vi "EncAlg.vi"(10 "EnValIn":dbl[](array[numeric]), 11 "element":T1) -> (0 "VelValOut":dbl[](array[numeric]), 1 "0, 1":i16, 2 "logical AND":bool)   [LabVIEW 2019]
panel:
  out "x":dbl
  out "y":dbl
  out "o":dbl
  out "Sense":dbl
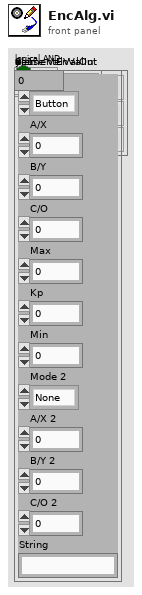
[diagram p1: front panel]
types:
  T1 = cluster{"Mode":enum16{"Button", "Encoder", "Delay", "IR Stop", "Line Stop"}, "A/X":dbl, "B/Y":dbl, "C/O":dbl, "Max":dbl, "Kp":dbl, "Min":dbl, "Mode 2":enum16{"None", "IR Stabilize", "Line Stabilize", "Encoder", "IR Stop", "Servo"}, "A/X 2":dbl, "B/Y 2":dbl, "C/O 2":dbl, "String":string}
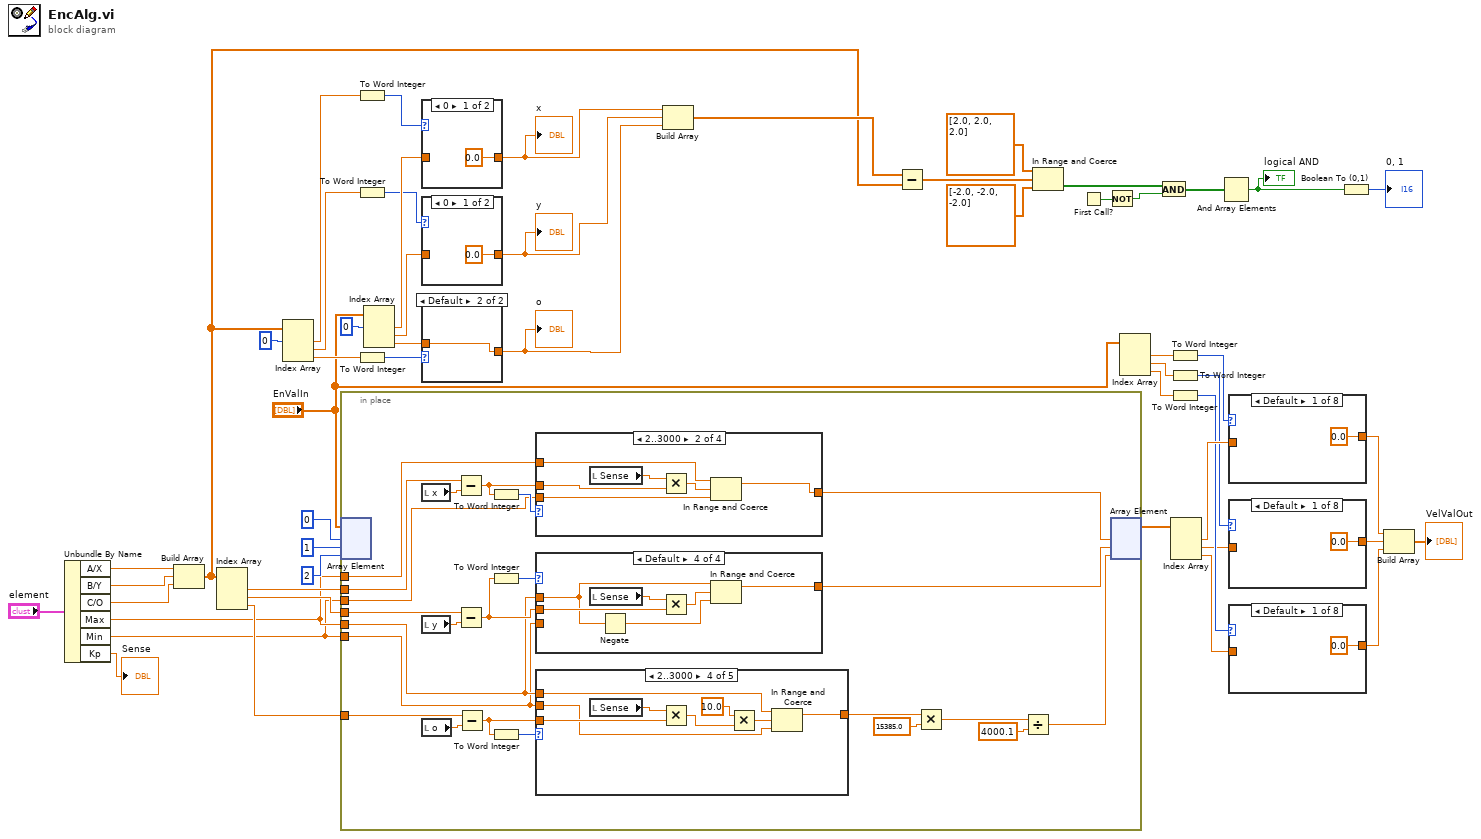
[diagram p0: block diagram]
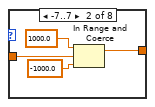
[diagram p2: hidden frame]
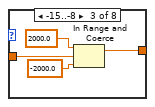
[diagram p3: hidden frame]
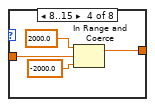
[diagram p4: hidden frame]
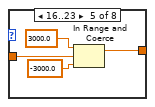
[diagram p5: hidden frame]
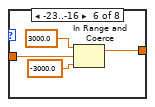
[diagram p6: hidden frame]
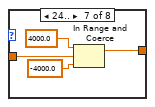
[diagram p7: hidden frame]
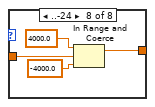
[diagram p8: hidden frame]
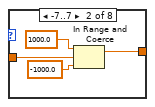
[diagram p9: hidden frame]
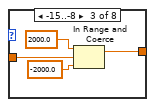
[diagram p10: hidden frame]
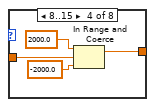
[diagram p11: hidden frame]
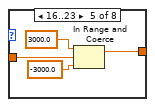
[diagram p12: hidden frame]
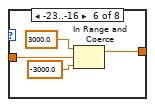
[diagram p13: hidden frame]
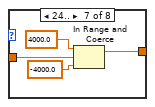
[diagram p14: hidden frame]
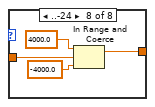
[diagram p15: hidden frame]
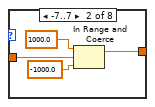
[diagram p16: hidden frame]
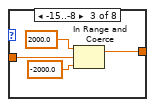
[diagram p17: hidden frame]
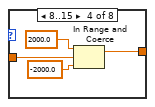
[diagram p18: hidden frame]
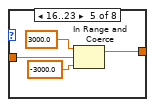
[diagram p19: hidden frame]
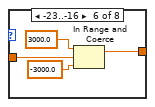
[diagram p20: hidden frame]
diagram:
  n1 = Unbundle By Name("element") -> ("A/X"=w47:dbl, "B/Y"=w46:dbl, "C/O"=w45:dbl, "Max"=w44:dbl, "Min"=w43:dbl, "Kp"=→"Sense":dbl)
  n2 = Build Array(w47, w46, w45) -> (w1:dbl[])
  n3 = Index Array(array=w1) -> (element #1=w49:dbl, element #2=w53:dbl, element #3=w48:dbl)  [unwired: 3 in]
  n4 = Index Array(array=w1, index #1=0 ("index")) -> (element #1=w39:dbl, element #2=w38:dbl, element #3=w37:dbl)  [unwired: 2 in]
  n5 = in-place {
    in-place-border: w53 -> [w76]
    in-place-border: w49 -> [w75]
    in-place-border: w48 -> [w74]
    in-place-border: w44 -> [w68]
    in-place-border: w43 -> [w67]
    in-place-border: w44 -> [w64]
    in-place-border: w43 -> [w63]
    n6 = in-place-array #1("EnValIn", 0, 1, 2) -> ()  [unwired: 3 out]
    n7 = local read "x"() -> (w54:dbl)
    n8 = local read "y"() -> (w55:dbl)
    n9 = local read "o"() -> (w56:dbl)
    n10 = Subtract(x=w75, y=w54) -> (x-y=w66:dbl)
    n11 = Subtract(x=w76, y=w55) -> (x-y=w65:dbl)
    n12 = Subtract(x=w74, y=w56) -> (x-y=w62:dbl)
    n13 = To Word Integer(number=w66) -> (16bit integer=w69:i16)
    n14 = To Word Integer(number=w65) -> (16bit integer=w70:i16)
    n15 = To Word Integer(number=w62) -> (16bit integer=w71:i16)
    n16 = case shown="2..3000" w69 {
      tunnel: w66 -> [_ w138 w146 w152]
      tunnel: [0.0 ("x") w139 w147 w153] -> w73
      tunnel: w68 -> [_ w137 w145 w151]
      tunnel: w67 -> [_ w136 w143 _]
      frame -1..1 {
      }
      frame 2..3000 {
        n17 = local read "Sense"() -> (w135:dbl)
        n18 = Multiply(x=w135, y=w138) -> (x*y=w140:dbl)
        n19 = In Range and Coerce(upper limit=w137, x=w140, lower limit=w136) -> (coerced(x)=w139:dbl)  [unwired: 1 out]
      }
      frame -3000..-2 {
        n20 = local read "Sense"() -> (w141:dbl)
        n21 = Negate(x=w143) -> (-x=w144:dbl)
        n22 = Negate(x=w145) -> (-x=w142:dbl)
        n23 = Multiply(x=w141, y=w146) -> (x*y=w148:dbl)
        n24 = In Range and Coerce(upper limit=w142, x=w148, lower limit=w144) -> (coerced(x)=w147:dbl)  [unwired: 1 out]
      }
      frame Default {
        n25 = local read "Sense"() -> (w149:dbl)
        n26 = Negate(x=w151) -> (-x=w150:dbl)
        n27 = Multiply(x=w149, y=w152) -> (x*y=w154:dbl)
        n28 = In Range and Coerce(upper limit=w151, x=w154, lower limit=w150) -> (coerced(x)=w153:dbl)  [unwired: 1 out]
      }
    }
    n29 = case shown="Default" w70 {
      tunnel: w65 -> [_ w117 w125 w131]
      tunnel: [0.0 ("x") w118 w126 w132] -> w72
      tunnel: w64 -> [_ w116 w121 w129]
      tunnel: w63 -> [_ w115 w122 _]
      frame -1..1 {
      }
      frame 2..3000 {
        n30 = local read "Sense"() -> (w114:dbl)
        n31 = Multiply(x=w114, y=w117) -> (x*y=w119:dbl)
        n32 = In Range and Coerce(upper limit=w116, x=w119, lower limit=w115) -> (coerced(x)=w118:dbl)  [unwired: 1 out]
      }
      frame -3000..-2 {
        n33 = local read "Sense"() -> (w120:dbl)
        n34 = Negate(x=w122) -> (-x=w123:dbl)
        n35 = Negate(x=w121) -> (-x=w124:dbl)
        n36 = Multiply(x=w120, y=w125) -> (x*y=w127:dbl)
        n37 = In Range and Coerce(upper limit=w124, x=w127, lower limit=w123) -> (coerced(x)=w126:dbl)  [unwired: 1 out]
      }
      frame Default {
        n38 = local read "Sense"() -> (w128:dbl)
        n39 = Negate(x=w129) -> (-x=w130:dbl)
        n40 = Multiply(x=w128, y=w131) -> (x*y=w133:dbl)
        n41 = In Range and Coerce(upper limit=w129, x=w133, lower limit=w130) -> (coerced(x)=w132:dbl)  [unwired: 1 out]
      }
    }
    n42 = case shown="2..3000" w71 {
      tunnel: w62 -> [w81 w90 _ w100 w110]
      tunnel: [w82 w91 0.0 ("x") w101 w111] -> w58
      tunnel: w64 -> [w78 w86 _ w98 w108]
      tunnel: w63 -> [_ w87 _ w97 w107]
      frame -1, 1 {
        n43 = local read "Sense"() -> (w79:dbl)
        n44 = Negate(x=w78) -> (-x=w77:dbl)
        n45 = Multiply(x=w81, y=w79) -> (x*y=w80:dbl)
        n46 = Multiply(x=10.0, y=w80) -> (x*y=w84:dbl)
        n47 = In Range and Coerce(upper limit=w78, x=w84, lower limit=w77) -> (coerced(x)=w82:dbl)  [unwired: 1 out]
      }
      frame Default {
        n48 = local read "Sense"() -> (w88:dbl)
        n49 = Negate(x=w86) -> (-x=w85:dbl)
        n50 = Multiply(x=w90, y=w88) -> (x*y=w89:dbl)
        n51 = Multiply(x=10.0, y=w89) -> (x*y=w93:dbl)
        n52 = In Range and Coerce(upper limit=w87, x=w93, lower limit=w85) -> (coerced(x)=w91:dbl)  [unwired: 1 out]
      }
      frame 0 {
      }
      frame 2..3000 {
        n53 = local read "Sense"() -> (w99:dbl)
        n54 = Multiply(x=w99, y=w100) -> (x*y=w102:dbl)
        n55 = Multiply(x=10.0, y=w102) -> (x*y=w96:dbl)
        n56 = In Range and Coerce(upper limit=w98, x=w96, lower limit=w97) -> (coerced(x)=w101:dbl)  [unwired: 1 out]
      }
      frame -3000..-2 {
        n57 = local read "Sense"() -> (w109:dbl)
        n58 = Negate(x=w107) -> (-x=w105:dbl)
        n59 = Negate(x=w108) -> (-x=w106:dbl)
        n60 = Multiply(x=w109, y=w110) -> (x*y=w112:dbl)
        n61 = Multiply(x=10.0, y=w112) -> (x*y=w104:dbl)
        n62 = In Range and Coerce(upper limit=w106, x=w104, lower limit=w105) -> (coerced(x)=w111:dbl)  [unwired: 1 out]
      }
    }
    n63 = Multiply(x=w58, y=15385.0) -> (x*y=w61:dbl)
    n64 = Divide(x=w61, y=4000.1) -> (x/y=w57:dbl)
    n65 = in-place-array #1(w73, w72, w57) -> (w33:dbl[])  [unwired: 3 out]
  }
  n66 = To Word Integer(number=w39) -> (16bit integer=w18:i16)
  n67 = To Word Integer(number=w38) -> (16bit integer=w16:i16)
  n68 = To Word Integer(number=w37) -> (16bit integer=w15:i16)
  n69 = Index Array(array="EnValIn", index #1=0 ("index")) -> (element #1=w17:dbl, element #2=w36:dbl, element #3=w35:dbl)  [unwired: 2 in]
  n70 = case shown="0" w18 {
    tunnel: [0.0 w156] -> w5
    tunnel: w17 -> [_ w156]
    frame 0 {
    }
    frame Default {
    }
  }
  "x" <- w5
  n71 = case shown="0" w16 {
    tunnel: [0.0 w158] -> w4
    tunnel: w36 -> [_ w158]
    frame 0 {
    }
    frame Default {
    }
  }
  "y" <- w4
  n72 = case shown="Default" w15 {
    tunnel: [0.0 w160] -> w3
    tunnel: w35 -> [_ w160]
    frame 0 {
    }
    frame Default {
    }
  }
  "o" <- w3
  n73 = Build Array(w5, w4, w3) -> (w2:dbl[])
  n74 = Subtract(x=w2, y=w1) -> (x-y=w14:dbl[])
  n75 = In Range and Coerce(upper limit=dbl[] [2.0, 2.0, 2.0], x=w14, lower limit=dbl[] [-2.0, -2.0, -2.0]) -> (In Range?=w11:bool[])  [unwired: 1 out]
  n76 = First Call?() -> (First Call?: T/F=w10:bool)
  n77 = Not(x=w10) -> (.not. x?=w9:bool)
  n78 = Index Array(array="EnValIn") -> (element #1=w30:dbl, element #2=w27:dbl, element #3=w26:dbl)  [unwired: 3 in]
  n79 = And(x=w11, y=w9) -> (x .and. y?=w8:bool[])
  n80 = To Word Integer(number=w30) -> (16bit integer=w29:i16)
  n81 = To Word Integer(number=w27) -> (16bit integer=w25:i16)
  n82 = To Word Integer(number=w26) -> (16bit integer=w24:i16)
  n83 = Index Array(array=w33) -> (element #1=w32:dbl, element #2=w23:dbl, element #3=w22:dbl)  [unwired: 3 in]
  n84 = And Array Elements(Boolean array=w8) -> (logical AND=w7:bool)
  "logical AND" <- w7
  n85 = case shown="Default" w29 {
    tunnel: w32 -> [_ w164 w168 w172 w176 w180 w184 w188]
    tunnel: [0.0 ("upper limit") w162 w166 w170 w174 w178 w182 w186] -> w28
    frame Default {
    }
    frame -7..7 {
      n86 = In Range and Coerce(upper limit=1000.0, x=w164, lower limit=-1000.0) -> (coerced(x)=w162:dbl)  [unwired: 1 out]
    }
    frame -15..-8 {
      n87 = In Range and Coerce(upper limit=2000.0, x=w168, lower limit=-2000.0) -> (coerced(x)=w166:dbl)  [unwired: 1 out]
    }
    frame 8..15 {
      n88 = In Range and Coerce(upper limit=2000.0, x=w172, lower limit=-2000.0) -> (coerced(x)=w170:dbl)  [unwired: 1 out]
    }
    frame 16..23 {
      n89 = In Range and Coerce(upper limit=3000.0, x=w176, lower limit=-3000.0) -> (coerced(x)=w174:dbl)  [unwired: 1 out]
    }
    frame -23..-16 {
      n90 = In Range and Coerce(upper limit=3000.0, x=w180, lower limit=-3000.0) -> (coerced(x)=w178:dbl)  [unwired: 1 out]
    }
    frame 24.. {
      n91 = In Range and Coerce(upper limit=4000.0, x=w184, lower limit=-4000.0) -> (coerced(x)=w182:dbl)  [unwired: 1 out]
    }
    frame ..-24 {
      n92 = In Range and Coerce(upper limit=4000.0, x=w188, lower limit=-4000.0) -> (coerced(x)=w186:dbl)  [unwired: 1 out]
    }
  }
  n93 = case shown="Default" w25 {
    tunnel: w23 -> [_ w193 w197 w201 w205 w209 w213 w217]
    tunnel: [0.0 ("upper limit") w191 w195 w199 w203 w207 w211 w215] -> w20
    frame Default {
    }
    frame -7..7 {
      n94 = In Range and Coerce(upper limit=1000.0, x=w193, lower limit=-1000.0) -> (coerced(x)=w191:dbl)  [unwired: 1 out]
    }
    frame -15..-8 {
      n95 = In Range and Coerce(upper limit=2000.0, x=w197, lower limit=-2000.0) -> (coerced(x)=w195:dbl)  [unwired: 1 out]
    }
    frame 8..15 {
      n96 = In Range and Coerce(upper limit=2000.0, x=w201, lower limit=-2000.0) -> (coerced(x)=w199:dbl)  [unwired: 1 out]
    }
    frame 16..23 {
      n97 = In Range and Coerce(upper limit=3000.0, x=w205, lower limit=-3000.0) -> (coerced(x)=w203:dbl)  [unwired: 1 out]
    }
    frame -23..-16 {
      n98 = In Range and Coerce(upper limit=3000.0, x=w209, lower limit=-3000.0) -> (coerced(x)=w207:dbl)  [unwired: 1 out]
    }
    frame 24.. {
      n99 = In Range and Coerce(upper limit=4000.0, x=w213, lower limit=-4000.0) -> (coerced(x)=w211:dbl)  [unwired: 1 out]
    }
    frame ..-24 {
      n100 = In Range and Coerce(upper limit=4000.0, x=w217, lower limit=-4000.0) -> (coerced(x)=w215:dbl)  [unwired: 1 out]
    }
  }
  n101 = case shown="Default" w24 {
    tunnel: w22 -> [_ w222 w226 w230 w234 w238 w242 w246]
    tunnel: [0.0 ("upper limit") w220 w224 w228 w232 w236 w240 w244] -> w19
    frame Default {
    }
    frame -7..7 {
      n102 = In Range and Coerce(upper limit=1000.0, x=w222, lower limit=-1000.0) -> (coerced(x)=w220:dbl)  [unwired: 1 out]
    }
    frame -15..-8 {
      n103 = In Range and Coerce(upper limit=2000.0, x=w226, lower limit=-2000.0) -> (coerced(x)=w224:dbl)  [unwired: 1 out]
    }
    frame 8..15 {
      n104 = In Range and Coerce(upper limit=2000.0, x=w230, lower limit=-2000.0) -> (coerced(x)=w228:dbl)  [unwired: 1 out]
    }
    frame 16..23 {
      n105 = In Range and Coerce(upper limit=3000.0, x=w234, lower limit=-3000.0) -> (coerced(x)=w232:dbl)  [unwired: 1 out]
    }
    frame -23..-16 {
      n106 = In Range and Coerce(upper limit=3000.0, x=w238, lower limit=-3000.0) -> (coerced(x)=w236:dbl)  [unwired: 1 out]
    }
    frame 24.. {
      n107 = In Range and Coerce(upper limit=4000.0, x=w242, lower limit=-4000.0) -> (coerced(x)=w240:dbl)  [unwired: 1 out]
    }
    frame ..-24 {
      n108 = In Range and Coerce(upper limit=4000.0, x=w246, lower limit=-4000.0) -> (coerced(x)=w244:dbl)  [unwired: 1 out]
    }
  }
  n109 = Boolean To (0,1)(Boolean=w7) -> (0, 1=→"0, 1":i16)
  n110 = Build Array(w28, w20, w19) -> (→"VelValOut":dbl[])
